vi "InitialTest.vi"() -> ()   [LabVIEW 2016]
panel:
  out "Boolean":bool
  in  "Number 2":dbl
  in  "Number 1":dbl
  in  "String":string
  in  "N2":dbl
  in  "N1":dbl
  out "Boolean 2":bool
  out "Y":dbl
  in  "X":dbl
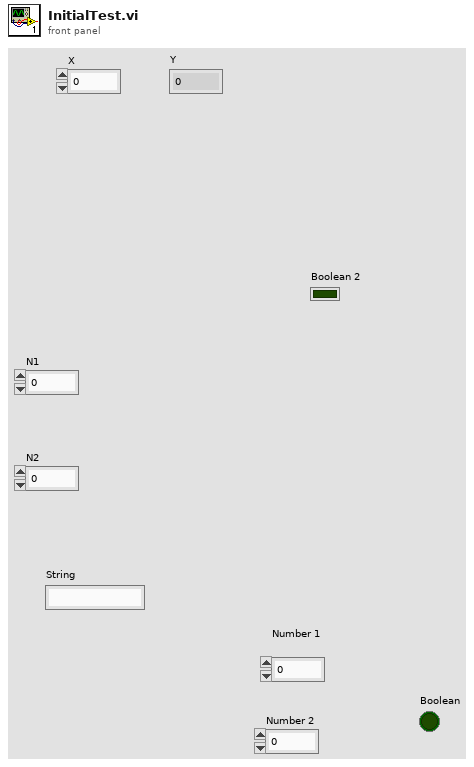
[diagram p1: front panel]
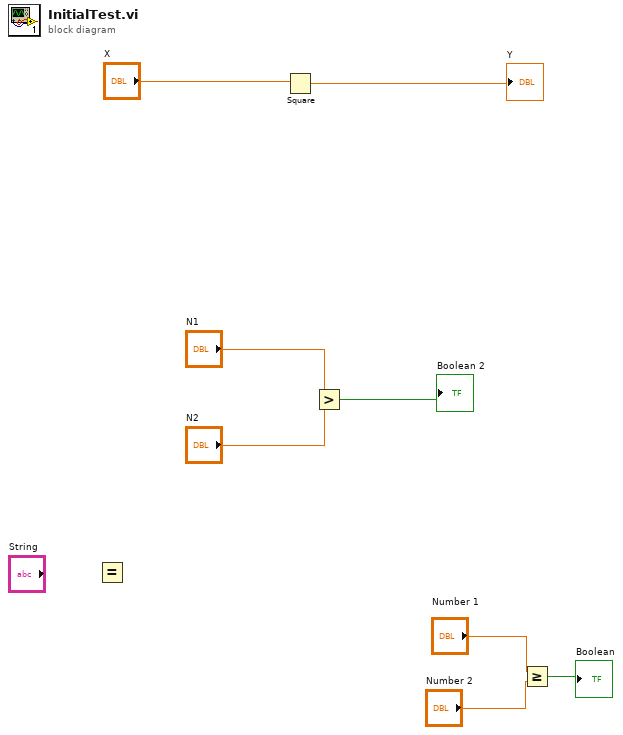
[diagram p0: block diagram]
diagram:
  n1 = Equal?() -> ()  [unwired: 2 in, 1 out]
  n2 = Square(x="X") -> (x^2=→"Y":dbl)
  n3 = Greater?(x="N1", y="N2") -> (0:→"Boolean 2":bool)
  n4 = Greater Or Equal?(x="Number 1", y="Number 2") -> (x >= y?=→"Boolean":bool)
